vi "close_data_log.vi"(8 "error in (no error)":errorcluster, 11 "raw_stream_logger in":refnum<class "raw_stream_logger.lvclass">) -> (0 "error out":errorcluster, 3 "raw_stream_logger out":refnum<class "raw_stream_logger.lvclass">)   [LabVIEW 2015, in "raw_stream_logger.lvclass"]
uses:
  raw_stream_logger.lvclass
  raw_stream_logger.lvclass/raw_stream_logger.ctl
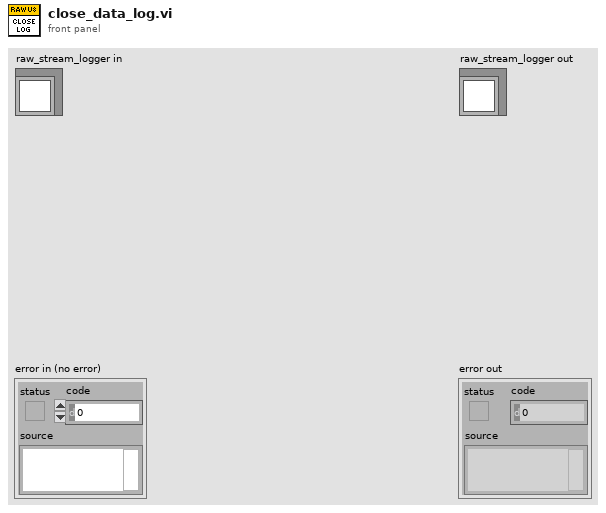
[diagram p1: front panel]
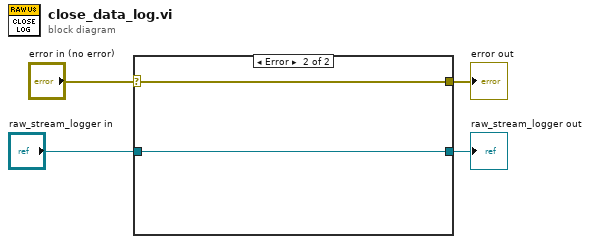
[diagram p0: block diagram]
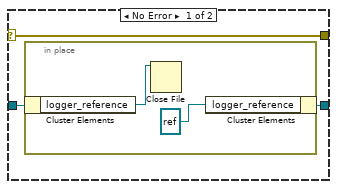
[diagram p2: hidden frame]
diagram:
  n1 = case shown="Error" "error in (no error)" {
    selector: "error in (no error)" -> [w5 w11]
    tunnel: "raw_stream_logger in" -> [w7 w10]
    tunnel: [w6 w10] -> w2
    tunnel: [w5 w11] -> w1
    frame No Error {
      n2 = in-place {
        n3 = in-place-cluster #1(w7) -> ("logger_reference"=w9:refnum<file>)
        n4 = Close File(refnum=w9) -> ()  [unwired: 1 in, 2 out]
        n5 = in-place-cluster #1("logger_reference"=refnum<file> refnum) -> (w6:refnum<class "raw_stream_logger.lvclass">)
      }
    }
    frame Error {
    }
  }
  "error out" <- w1
  "raw_stream_logger out" <- w2
